vi "Search and Match Towel to Design.vi"(10 "Towel":T4, 11 "Design Data":T1) -> (0 "Check If Full Out":bool, 3 "Design Array Out":T1[](array[typedef]))   [LabVIEW 2024]
uses:
  Cluster_Design Data.ctl
  ENUM_Stripe Select.ctl
  Cluster_Design Towel ID Data.ctl
  Cluster_Towel Data.ctl
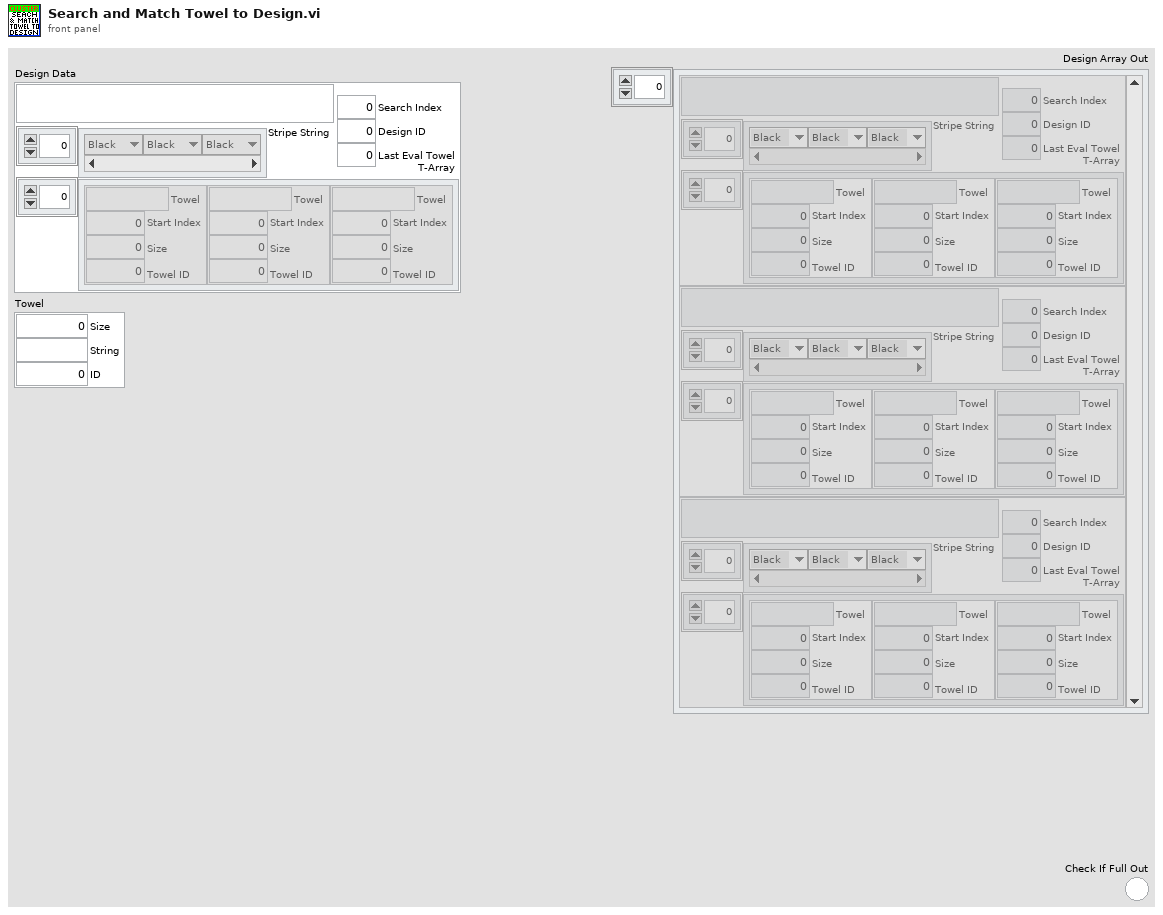
[diagram p1: front panel]
types:
  T1 = typedef "Cluster_Design Data.ctl" = cluster{"Stripe String":string, "Stripes":T2[], "T-Array":T3[], "Search Index":i32, "Design ID":i32, "Last Eval Towel":i32}
  T2 = typedef "ENUM_Stripe Select.ctl" = enum16{"Black", "Blue", "Green", "Red", "White"}
  T3 = typedef "Cluster_Design Towel ID Data.ctl" = cluster{"Towel":string, "Start Index":i32, "Size":i32, "Towel ID":i32}
  T4 = typedef "Cluster_Towel Data.ctl" = cluster{"Size":i32, "String":string, "ID":i32}
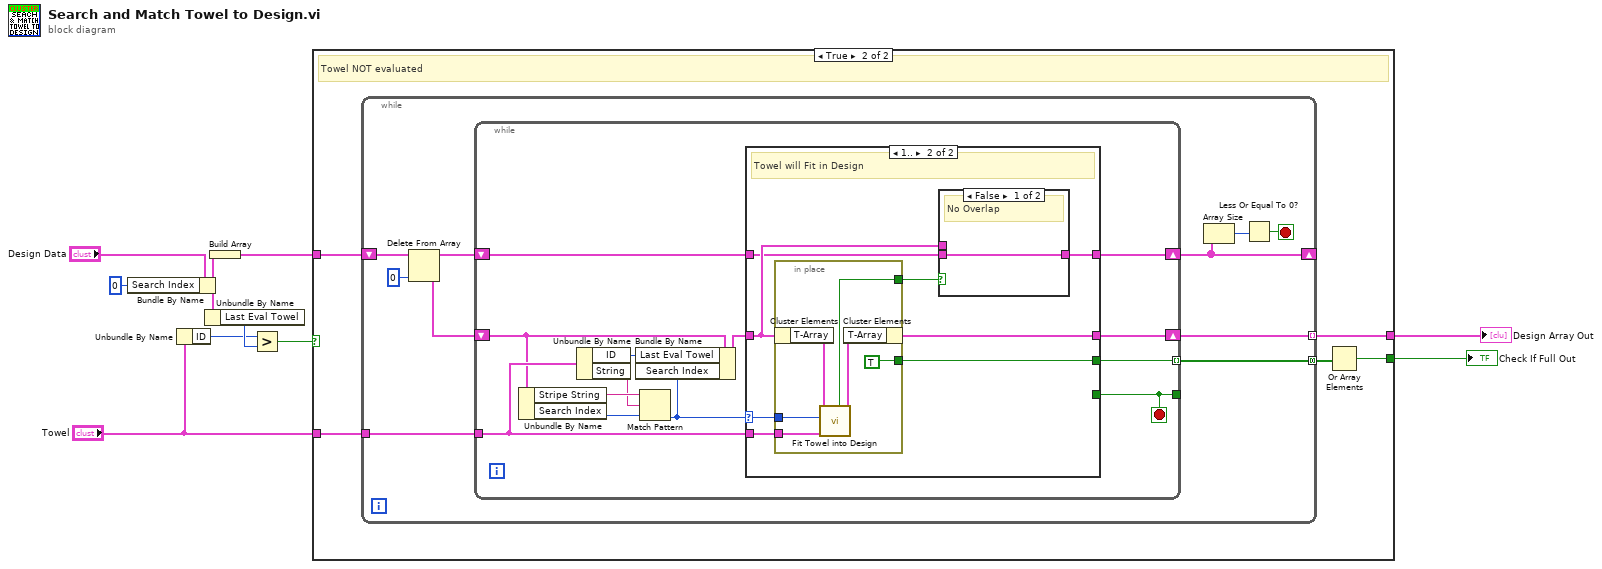
[diagram p0: block diagram]
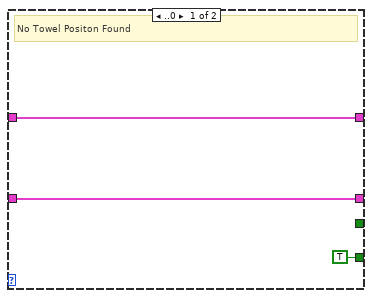
[diagram p3: hidden frame]
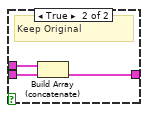
[diagram p4: hidden frame]
diagram:
  n1 = Bundle By Name(cluster="Design Data", "Search Index"=0) -> (w3:T1)
  n2 = Unbundle By Name("Towel") -> ("ID"=w6:i32)
  n3 = Unbundle By Name(w3) -> ("Last Eval Towel"=w7:i32)
  n4 = Build Array(w3) -> (w2:T1[])
  n5 = Greater?(x=w6, y=w7) -> (0:w1:bool)
  n6 = case shown="True" w1 {
    tunnel: [_ w15] -> w8
    tunnel: w2 -> [w11 w12]
    tunnel: "Towel" -> [_ w14]
    tunnel: [w11 w13] -> w4
    frame False {
      # "Towel Already Evaluated"
    }
    frame True {
      # "Towel NOT evaluated"
      n7 = while {
        tunnel: w14 -> [w26]
        shift-right: [w19] -> _
        shift-left: w12 -> [w25]
        tunnel: [w18] -> w13 mode=indexing
        tunnel: [w17] -> w16 mode=concatenating
        stop <- w20 stop-if-true
        n8 = Delete From Array(array=w25, index=0) -> (deleted portion=w22:T1, array with subset deleted=w24:T1[])  [unwired: 1 in]
        n9 = while {
          tunnel: w26 -> [w35]
          shift-right: [w37] -> w19
          shift-left: w24 -> [w39]
          shift-right: [w38] -> w18
          shift-left: w22 -> [w34]
          tunnel: [w36] -> _
          tunnel: [w33] -> w17 mode=indexing
          stop <- w36 stop-if-true
          n10 = Unbundle By Name(w34) -> ("Stripe String"=w32:string, "Search Index"=w30:i32)
          n11 = Unbundle By Name(w35) -> ("ID"=w28:i32, "String"=w27:string)
          n12 = Match Pattern(string=w32, regular expression=w27, offset (0)=w30) -> (offset past match=w29:i32)  [unwired: 3 out]
          n13 = Bundle By Name(cluster=w34, "Last Eval Towel"=w28, "Search Index"=w29) -> (w31:T1)
          n14 = case shown="1.." w29 {
            selector: w29 -> [_ w50]
            tunnel: w31 -> [w42 w48]
            tunnel: [w42 w49] -> w38
            tunnel: w35 -> [_ w44]
            tunnel: w39 -> [w40 w47]
            tunnel: [w40 w46] -> w37
            tunnel: [TRUE _] -> w36
            tunnel: [_ w45] -> w33
            frame ..0 {
              # "No Towel Positon Found"
            }
            frame 1.. {
              # "Towel will Fit in Design"
              n15 = in-place {
                in-place-border: w50 -> [w54]
                in-place-border: [TRUE] -> w45
                in-place-border: w44 -> [w53]
                in-place-border: [w51] -> w43
                n16 = in-place-cluster #1(w48) -> ("T-Array"=w56:T3[])
                n17 = call "Fit Towel into Design.vi"("Towel"=w53, "Offset Past Match"=w54, "T-Array"=w56) -> ("T-Array Out"=w55:T3[], "Keep Original Out"=w51:bool)  [unwired: 7 in]
                n18 = in-place-cluster #1("T-Array"=w55) -> (w49:T1)
              }
              n19 = case shown="False" w43 {
                tunnel: w48 -> [_ w58]
                tunnel: w47 -> [w57 w60]
                tunnel: [w57 w59] -> w46
                frame False {
                  # "No Overlap"
                }
                frame True {
                  # "Keep Original"
                  n20 = Build Array (concatenate)(w58, w60) -> (w59:T1[])
                }
              }
            }
          }
        }
        n21 = Array Size(array=w19) -> (size(s)=w21:i32)
        n22 = Less Or Equal To 0?(x=w21) -> (x <= 0?=w20:bool)
      }
      n23 = Or Array Elements(Boolean array=w16) -> (logical OR=w15:bool)
    }
  }
  "Check If Full Out" <- w8
  "Design Array Out" <- w4
